vi "Create Configured Instr from JSON.vi"(8 "error in (no error)":errorcluster, 11 "<JSON CFG>":string) -> (0 "error out":errorcluster, 2 "IInstrument Base":refnum<class "Instrument.lvclass">)   [LabVIEW 2023, in "HAL GOOP4.lvlib" / "Measure and Stimulus Subsystems.lvclass"]
uses:
  Measure and Stimulus Subsystems.lvclass
  Instrument/Instrument.lvclass
  Configuration/Configuration JSON/Configuration JSON Base/CFG JSON.lvclass
  30f21247-d589-44c2-bdab-c07647d922d1.vi
  <vilib>/JDP Science/JSONtext/Find Item.vi
  <vilib>/JDP Science/JSONtext/Next JSON Value.vi
  <vilib>/JDP Science/JSONtext/String Subset.vi
  <vilib>/JDP Science/JSONtext/Parsing/Advance past next JSON Value (inlined COPY).vi
  <vilib>/JDP Science/JSONtext/Parsing/Advance past whitespace.vi
  <vilib>/JDP Science/JSONtext/Parsing/Advance past String.vi
  <vilib>/JDP Science/JSONtext/Parsing/Advance past Number.vi
  <vilib>/JDP Science/JSONtext/Parsing/Advance past Line Ending.vi
  <vilib>/JDP Science/JSONtext/Parsing/Parse Full Path or Item Name.vi
  <vilib>/JDP Science/JSONtext/Parsing/Advance past Array.vi
  <vilib>/JDP Science/JSONtext/Parsing/Advance past Object.vi
  <vilib>/JDP Science/JSONtext/support/Error Cluster From Code.vi
  <vilib>/JDP Science/JSONtext/Offset/Find Item Locations by Path.vi
  <vilib>/JDP Science/JSONtext/JSON text to Variant.vi
  <vilib>/Utility/error.llb/Error Cluster From Error Code.vi
  <vilib>/JDP Science/JSONtext/LVClass Serializer/JSONtext LVClass Serializer.lvclass
  <vilib>/ErrorRing/Error Ring.xnode
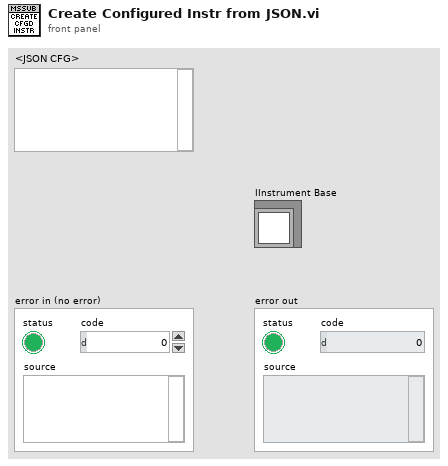
[diagram p1: front panel]
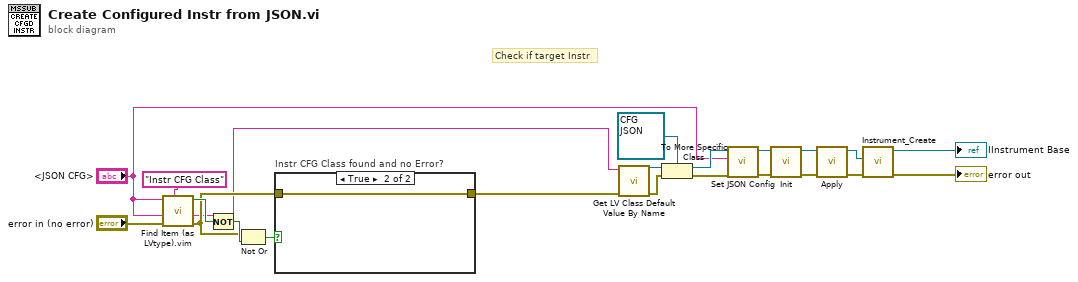
[diagram p0: block diagram]
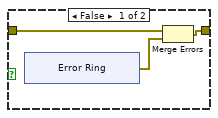
[diagram p2: hidden frame]
diagram:
  # "Check if target Instr"
  n1 = call "Find Item (as LVtype).vim"("$Path or Item Name"="Instr CFG Class", "error in (no error)"="error in (no error)", "Data Type and Default Value"="<JSON CFG>", "JSON"="<JSON CFG>") -> ("error out"=w17:errorcluster, "Data"=w11:string, "Found"=w19:bool)  [unwired: 4 in, 1 out]
  n2 = Not(x=w19) -> (.not. x?=w21:bool)
  n3 = Not Or(1:w21, 2:w17) -> (0:w20:bool)
  n4 = case "Instr CFG Class found and no Error?" shown="True" w20 {
    tunnel: [w25 w31] -> w18
    tunnel: w17 -> [w23 w31]
    frame False {
      n5 = xnode "Error Ring"() -> ("error out"=w24:errorcluster)
      n6 = Merge Errors(w23, w24) -> (w25:errorcluster)
    }
    frame True {
    }
  }
  n7 = call <vilib>:"Get LV Class Default Value By Name.vi"("error in (no error)"=w18, "class name"=w11) -> ("error out"=w14:errorcluster, "object"=w13:refnum<class>)  [unwired: 8 in]
  n8 = To More Specific Class(target class=refnum<class "CFG JSON.lvclass"> refnum ("HAL GOOP4.lvlib:CFG JSON Base.lvclass"), reference=w13, error in=w14) -> (specific class reference=w10:refnum<class "CFG JSON.lvclass">, error out=w9:errorcluster)
  n9 = call "Set JSON Config.vi"("error in (no error)"=w9, "<JSON>Config>"="<JSON CFG>", "CFG Base in"=w10) -> ("error out"=w15:errorcluster, "CFG Base out"=w4:refnum<class "CFG JSON.lvclass">)  [unwired: 7 in]
  n10 = call-dynamic "Init.vi"("error in (no error)"=w15, "IConfigure in"=w4) -> ("error out"=w5:errorcluster, "IConfigure out"=w2:refnum<class "CFG JSON.lvclass">)  [unwired: 8 in]
  n11 = call-dynamic "Apply.vi"("error in (no error)"=w5, "IConfigure in"=w2) -> ("error out"=w3:errorcluster, "IConfigure out"=w1:refnum<class "CFG JSON.lvclass">)  [unwired: 8 in]
  n12 = call "Instrument_Create.vi"("Error In"=w3, "IConfigure"=w1) -> ("Error Out"=→"error out":errorcluster, "reference out"=→"IInstrument Base":refnum<class "Instrument.lvclass">)  [unwired: 8 in]
